vi "Discrete-Acquisition-Signal-Path.vi"() -> ()   [LabVIEW 2020]
uses:
  <vilib>/SLSC/Initialize Session with Devices.vi
  <vilib>/SLSC/Set Phys Chan Property (1D I32).vi
  <vilib>/SLSC/Set Phys Chan Property (Bool).vi
  <vilib>/SLSC/Set Phys Chan Property (I32).vi
  <vilib>/SLSC/Set Phys Chan Property (DBL).vi
  <vilib>/SLSC/Commit Properties for Devices.vi
  <vilib>/SLSC/Close Session.vi
  <vilib>/SLSC/SLSC.lvlib
  <vilib>/SLSC_Switch/SLSC Switch.lvlib
  <vilib>/SLSC_Switch/Initialize with Topology (Override Switches).vi
panel:
  in  "2010 Module":refnum<k21>="SET-2010-Mod2"
  in  "Bank 0 Pullup Enable":bool=TRUE
  in  "Bank 0 Vsup":i32(ring) items=["Vsup_Off", "Vsup_0", "Vsup_1"]
  in  "Bank 0 Input Threshold (V)":dbl=0.74 min=0.74 max=5.2
  in  "Bank 0 5 V Range Enable":bool=TRUE
  in  "Bank 0 Configuration":i32[](array[ring])=[0, 0, 0, 0] items=["Input", "Output_Source", "Output_Sink", "Output_PushPull"]
  in  "Enable Channels":bool=TRUE
  in  "12201 Module":refnum<k21>="SLSC-12001-xxxxxxxx-Mod1"
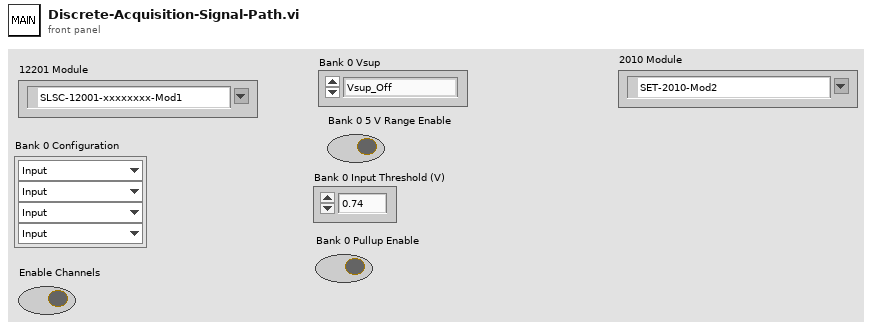
[diagram p1: front panel]
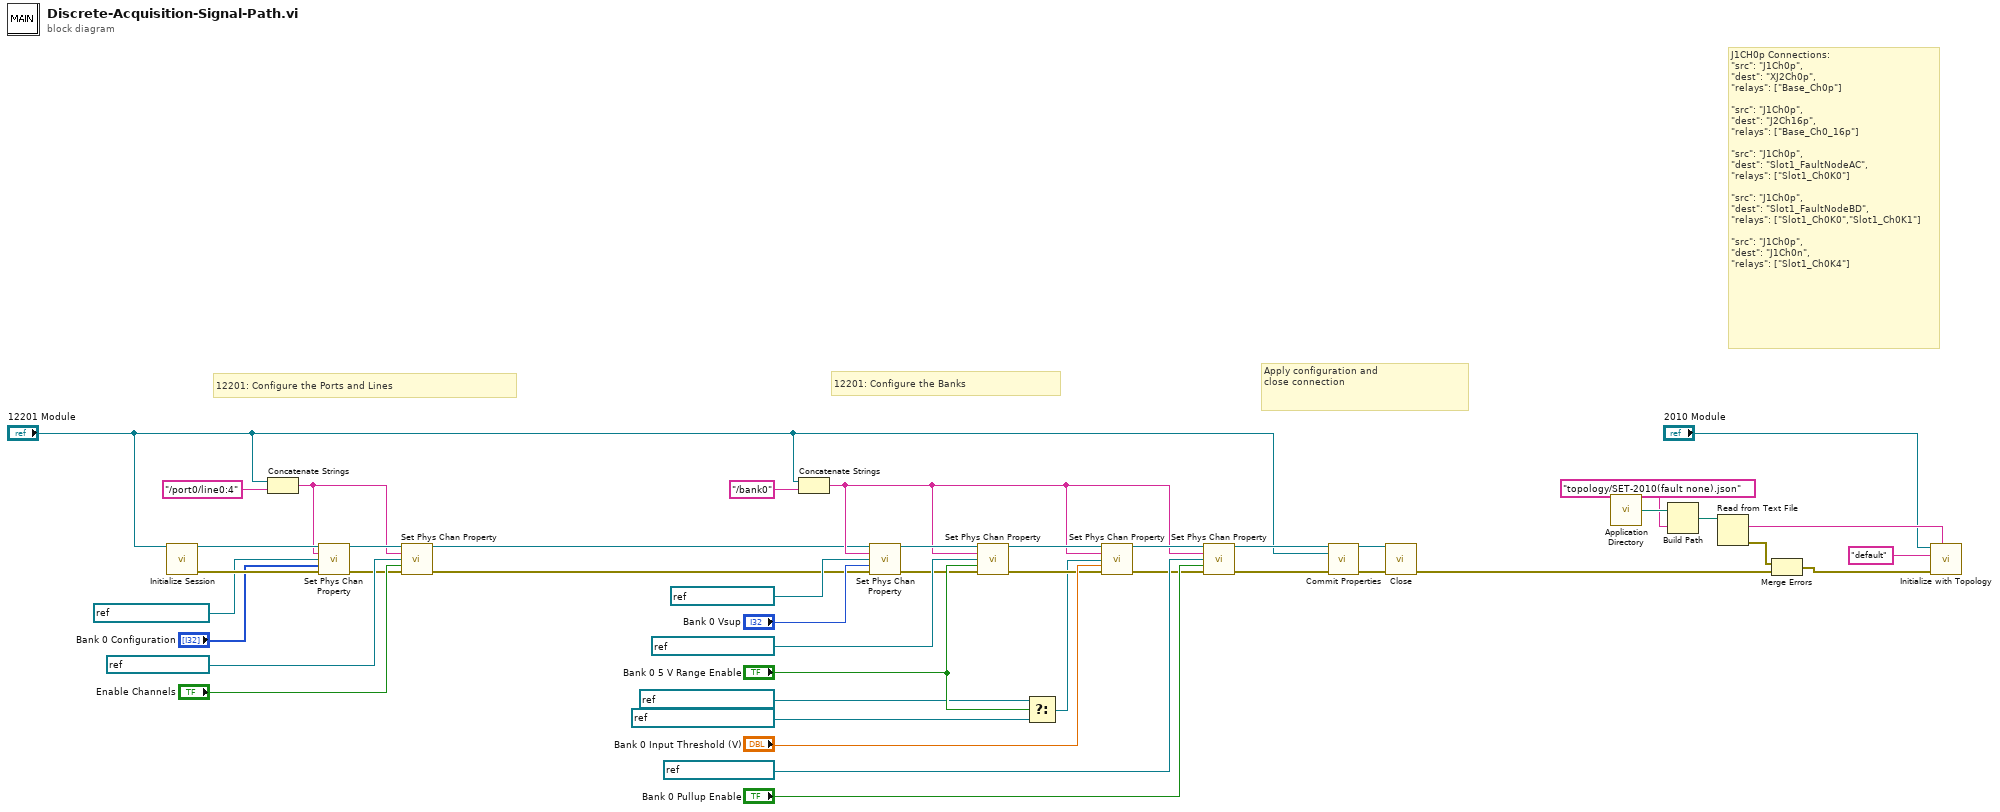
[diagram p0: block diagram]
diagram:
  # "J1CH0p Connections:\n\"src\": \"J1Ch0p\",\n\"dest\": \"XJ2Ch0p\",\n\"relays\": [\"Base_Ch0p\"]\n\n\"src\": \"J1Ch0p\",\n\"dest\": \"J2Ch16p\",\n\"relays\": [\"Base_Ch0_16p\"]\n\n\"src\": \"J1Ch0p\",\n\"dest\": \"Slot1_FaultNodeAC\",\n\"relays\": [\"Slot1_Ch0K0\"]\n\n\"src\": \"J1Ch0p\",\n\"dest\": \"Slot1_FaultNodeBD\",\n\"relays\": [\"Slot1_Ch0K0\",\"Slot1_Ch0K1\"]\n\n\"src\": \"J1Ch0p\",\n\"dest\": \"J1Ch0n\",\n\"relays\": [\"Slot1_Ch0K4\"]"
  # "Apply configuration and \nclose connection"
  # "12201: Configure the Ports and Lines"
  # "12201: Configure the Banks"
  n1 = call-poly <vilib>:"Initialize Session.vi"("devices"="12201 Module") -> ("session out"=w43:refnum<k21>, "error out"=w44:errorcluster)  [unwired: 13 in]
  n2 = Concatenate Strings("12201 Module", "/port0/line0:4") -> (w37:string)
  n3 = call-poly <vilib>:"Set Phys Chan Property.vi"("session in"=w43, "physical channels"=w37, "property"=refnum<k21> "NI.Line.Direction", "property value"="Bank 0 Configuration", "error in (no error)"=w44) -> ("session out"=w39:refnum<k21>, "error out"=w38:errorcluster)  [unwired: 9 in]
  n4 = call-poly <vilib>:"Set Phys Chan Property.vi"("session in"=w39, "physical channels"=w37, "property"=refnum<k21> "NI.Line.Enable", "property value"="Enable Channels", "error in (no error)"=w38) -> ("session out"=w15:refnum<k21>, "error out"=w25:errorcluster)  [unwired: 9 in]
  n5 = Concatenate Strings("12201 Module", "/bank0" ("string")) -> (w18:string)
  n6 = call-poly <vilib>:"Set Phys Chan Property.vi"("session in"=w15, "physical channels"=w18, "property"=refnum<k21> "NI.VsupSelect", "property value"="Bank 0 Vsup", "error in (no error)"=w25) -> ("session out"=w20:refnum<k21>, "error out"=w19:errorcluster)  [unwired: 9 in]
  n7 = call-poly <vilib>:"Set Phys Chan Property.vi"("session in"=w20, "physical channels"=w18, "property"=refnum<k21> "NI.RangeEnable5V", "property value"="Bank 0 5 V Range Enable", "error in (no error)"=w19) -> ("session out"=w22:refnum<k21>, "error out"=w21:errorcluster)  [unwired: 9 in]
  n8 = Select(t=refnum<k21> "NI.InputThreshold5V" ("property"), s="Bank 0 5 V Range Enable", f=refnum<k21> "NI.InputThreshold33V" ("property")) -> (s? t:f=w17:refnum<k21>)
  n9 = call-poly <vilib>:"Set Phys Chan Property.vi"("session in"=w22, "physical channels"=w18, "property"=w17, "property value"="Bank 0 Input Threshold (V)", "error in (no error)"=w21) -> ("session out"=w24:refnum<k21>, "error out"=w23:errorcluster)  [unwired: 9 in]
  n10 = call-poly <vilib>:"Set Phys Chan Property.vi"("session in"=w24, "physical channels"=w18, "property"=refnum<k21> "NI.PullupEnable", "property value"="Bank 0 Pullup Enable", "error in (no error)"=w23) -> ("session out"=w14:refnum<k21>, "error out"=w12:errorcluster)  [unwired: 9 in]
  n11 = call-poly <vilib>:"Commit Properties.vi"("session in"=w14, "devices"="12201 Module", "error in (no error)"=w12) -> ("session out"=w10:refnum<k21>, "error out"=w11:errorcluster)  [unwired: 11 in]
  n12 = call-poly <vilib>:"Close.vi"("session in"=w10, "error in (no error)"=w11) -> ("error out"=w6:errorcluster)  [unwired: 13 in]
  n13 = call <vilib>:"Application Directory.vi"() -> ("Application Directory"=w9:path)
  n14 = Build Path(base path=w9, name or relative path="topology/SET-2010(fault none).json") -> (appended path=w7:path)
  n15 = Read from Text File(file (use dialog)=w7) -> (text=w3:string, error out=w4:errorcluster)  [unwired: 3 in, 2 out]
  n16 = Merge Errors(w4, w6) -> (w5:errorcluster)
  n17 = call-poly <vilib>:"Initialize with Topology.vi"("switches json"=w3, "error in (no error)"=w5, "topology"="default", "device"="2010 Module") -> ()  [unwired: 6 in, 2 out]
